vi "Draw.vi"(6 "Color Box":u32(colorbox), 8 "Error In":errorcluster, 9 "Offset":T1, 10 "Picture in":picture, 11 "Panel Object in":refnum<class "Panel Object.lvclass">) -> (0 "Error Out":errorcluster, 2 "Picture out":picture, 3 "Panel Object out":refnum<class "Panel Object.lvclass">)   [LabVIEW 2018, in "Panel Object.lvclass"]
uses:
  <resource>/dialog/QuickDrop/plugins/PaneRelief/Classes/Panel Object/Panel Object.lvclass
  <resource>/dialog/QuickDrop/plugins/PaneRelief/Typedefs/Point--Cluster.ctl
  <resource>/dialog/QuickDrop/plugins/PaneRelief/Classes/Panel Object/Panel Object.lvclass/Panel Object.ctl
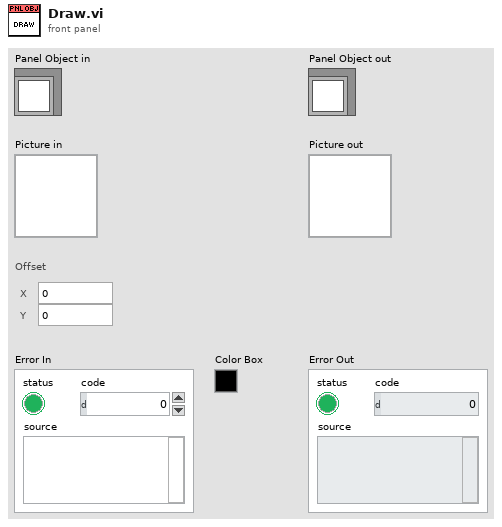
[diagram p1: front panel]
types:
  T1 = typedef "Point--Cluster.ctl" = cluster{"Horizontal":i32, "Vertical":i32}
  T2 = cluster{"left":i16, "top":i16, "right":i16, "bottom":i16}
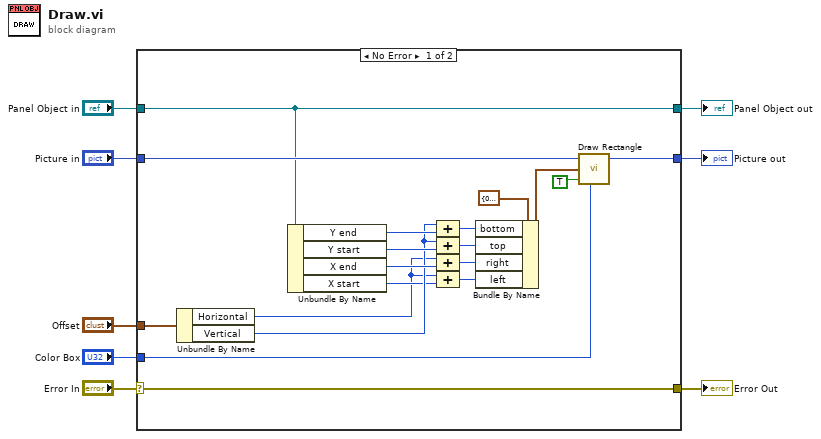
[diagram p0: block diagram]
diagram:
  n1 = case shown="No Error" "Error In" {
    selector: "Error In" -> [w27 w30]
    tunnel: [w27 w30] -> w5
    tunnel: [w13 w29] -> w7
    tunnel: "Panel Object in" -> [w13 w29]
    tunnel: "Picture in" -> [w16 w28]
    tunnel: [w15 w28] -> w3
    tunnel: "Offset" -> [w14 _]
    tunnel: "Color Box" -> [w12 _]
    frame No Error {
      n2 = Unbundle By Name(w14) -> ("Horizontal"=w9:i32, "Vertical"=w11:i32)
      n3 = Unbundle By Name(w13) -> ("Y end"=w23:i32, "Y start"=w22:i32, "X end"=w21:i32, "X start"=w10:i32)
      n4 = Compound Arithmetic op=ADD(w11, w23) -> (w20:i32)
      n5 = Compound Arithmetic op=ADD(w11, w22) -> (w19:i32)
      n6 = Compound Arithmetic op=ADD(w9, w21) -> (w18:i32)
      n7 = Compound Arithmetic op=ADD(w9, w10) -> (w17:i32)
      n8 = Bundle By Name(cluster=T2 {"left"=0, "top"=0, "right"=0, "bottom"=0} ("rect"), "bottom"=w20, "top"=w19, "right"=w18, "left"=w17) -> (w24:T2)
      n9 = call <vilib>:"Draw Rectangle.vi"("picture"=w16, "rect"=w24, "fill?(F)"=TRUE, "color(black)"=w12) -> ("new picture"=w15:picture)  [unwired: 5 in]
    }
    frame Error {
    }
  }
  "Panel Object out" <- w7
  "Error Out" <- w5
  "Picture out" <- w3
